vi "Subvi_Online_For_Offline_FBLDA_통합버전.vi"(0 "rate":dbl=500.0 caption="Rate" format="%0.2f", 1 "samples per channel":i32=25, 5 "Brain_data_source":dbl[][](array[numeric]) caption="EEG_Raw_Data" format="%0.3f", 7 "Target_Flash_Order":i64[][](array[numeric]), 8 "Value":T1, 9 "사용할 Parameter 갯수":i32=2, 10 "Weight":dbl[](array[numeric]), 11 "Path":path, 14 "Number":string, 16 "Matrix":T1, 17 "Channel selection":bool[](array[boolean])) -> (13 "LDA_Parameter":dbl[][](array[numeric]), 15 "EPR_발생_total":i16[](array[numeric]), 20 "output-0~8":i32, 22 "ERP_Parameters":dbl[][](array[numeric]))   [LabVIEW 2014]
uses:
  <vilib>/Analysis/Matrix/Datatypes/RealMatrix.ctl
  <vilib>/Analysis/3filter.llb/Filter Passband Type.ctl
  <vilib>/Analysis/baseanly.llb/Real A x B.vi
  <vilib>/Analysis/baseanly.llb/Mean (DBL).vi
  <vilib>/Analysis/3filter.llb/Butterworth Filter (DBL).vi
  <vilib>/Analysis/Matrix/Numeric/Conversions/Array To Matrix - RA.vi
  <vilib>/Analysis/Matrix/Numeric/Conversions/Array To Matrix - RA2.vi
  <vilib>/Analysis/Matrix/Numeric/Conversions/Matrix To Array - RM.vi
  <vilib>/Analysis/Matrix/Numeric/Multiply/Multiply - RM,RM.vi
  <vilib>/Analysis/Matrix/Numeric/Subtract/Subtract - RM,RM.vi
  <vilib>/Analysis/NI_AALBase.lvlib
  <vilib>/Analysis/Matrix/NI_Matrix.lvlib
  <vilib>/Utility/file.llb/Read From Spreadsheet File (DBL).vi
panel:
  out "최대값":dbl
  out "size(s)":i32[](array[numeric])
  out "A - B":T1
  out "Array 2":dbl[][](array[numeric])
  out "subarray":dbl[](array[numeric])
  out "Array":dbl[][](array[numeric])
  out "deleted portion":dbl[][](array[numeric])
  in  "LDA":path=path "C:/Users/Administrator/Desktop/공공복지안전사업연구-노수진/파일럿20130902/LDA_Matrix_Value.xls"
  out "#channel":i32
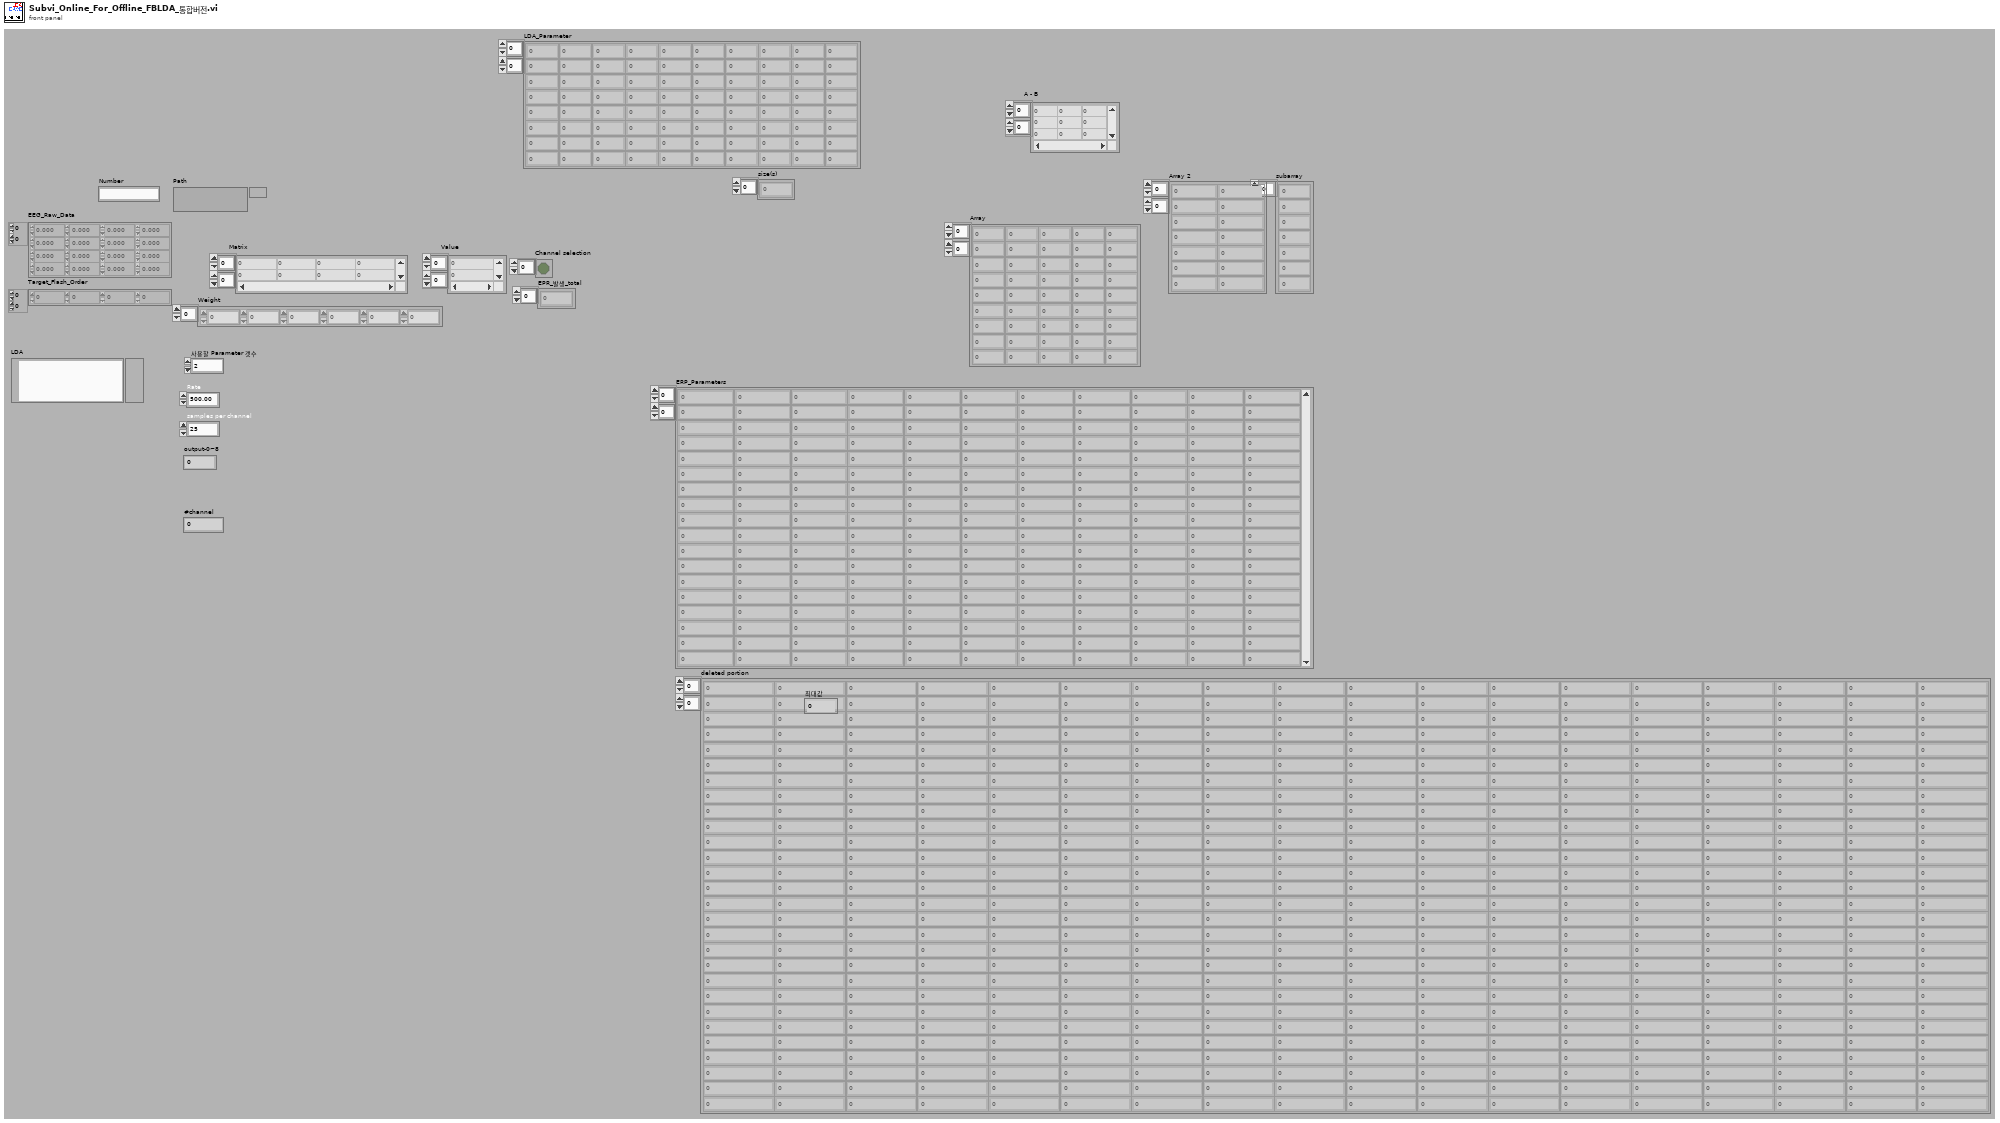
[diagram p1: front panel]
types:
  T1 = typedef "NI_Matrix.lvlib/RealMatrix.ctl" = dbl[][]
  T2 = typedef "NI_AALBase.lvlib/Filter Passband Type.ctl" = enum32{"Lowpass", "Highpass", "Bandpass", "Bandstop"}
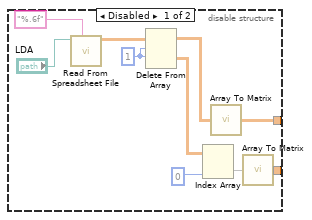
[diagram p3: hidden frame]
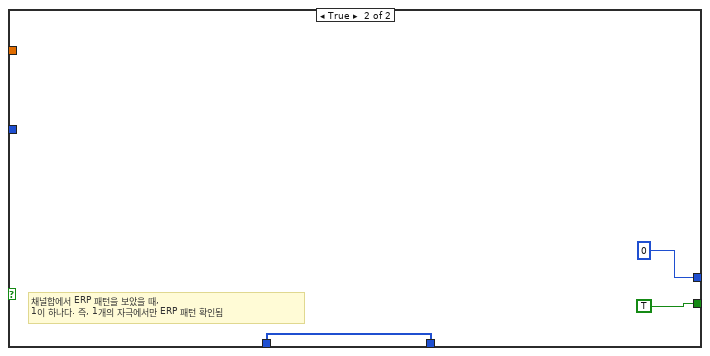
[diagram p4: hidden frame]
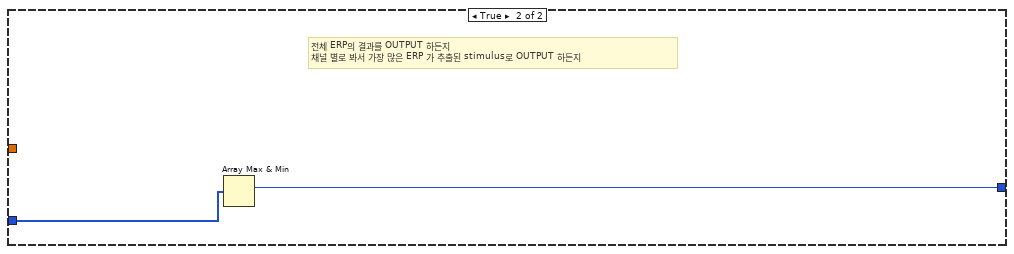
[diagram p5: hidden frame]
diagram:
  n1 = flat-sequence {
    tunnel: [w28] -> w23
    tunnel: [w52] -> w22
    tunnel: ["Target_Flash_Order"] -> w21
    tunnel: w23 -> [w52]
    tunnel: [w49] -> w20
    tunnel: w22 -> [w60]
    tunnel: w21 -> [w59]
    tunnel: w20 -> [w58]
    tunnel: [w53] -> w19
    tunnel: ["Weight"] -> w12
    tunnel: [w53] -> w1
    tunnel: w19 -> [w189]
    tunnel: [w191] -> w18
    tunnel: [w191] -> w17
    tunnel: [w191] -> w16
    tunnel: w12 -> [w186]
    tunnel: [w186] -> w11
    tunnel: [w180] -> w2
    tunnel: w1 -> [w180]
    tunnel: w18 -> [w228]
    tunnel: w17 -> [w234]
    tunnel: w16 -> [w221]
    tunnel: [w236] -> w15
    tunnel: w11 -> [w235]
    tunnel: [w235] -> w10
    tunnel: [w229] -> w9
    tunnel: [w219] -> w7
    tunnel: [w228] -> w5
    tunnel: [w227] -> w4
    tunnel: w2 -> [w220]
    tunnel: w15 -> [w257]
    tunnel: [w257] -> w14
    tunnel: w10 -> [_]
    tunnel: w9 -> [w260]
    tunnel: [w259] -> w8
    tunnel: w7 -> [w262]
    tunnel: [w262] -> w6
    tunnel: w5 -> [w261]
    tunnel: w4 -> [w258]
    tunnel: [w258] -> w3
    tunnel: [w285] -> w13
    tunnel: w14 -> [w286]
    tunnel: w8 -> [w284]
    tunnel: w6 -> [w283]
    tunnel: w3 -> [w282]
    tunnel: w13 -> [w307]
    frame #0 {
      n2 = Array Size(array="Brain_data_source") -> (size(s)=w29:i32[])
      n3 = Index Array(array=w29, index=1) -> (element=w31:i32)
      "#channel" <- w31
      n4 = for {
        N: w31 -> [_]
        tunnel: "Brain_data_source" -> [w36]
        shift-right: [w33] -> w25
        shift-left: dbl[][] [] ("Filtered X") -> [w34]
        tunnel: "Channel selection" -> [w32] mode=indexing
        i -> [w35]
        n5 = case shown="True" w32 {
          tunnel: w36 -> [_ w47]
          tunnel: w35 -> [_ w46]
          tunnel: w34 -> [w37 w40]
          tunnel: [w37 w39] -> w33
          frame False {
          }
          frame True {
            n6 = local read "rate"() -> (w41:dbl)
            n7 = Index Array(array=w47, index (col)=w46) -> (element=w45:dbl[])  [unwired: 1 in]
            n8 = call-poly <vilib>:"Butterworth Filter.vi"("filter type"=Filter_Passband_Type."Bandpass", "low cutoff freq: fl"=0.5, "high cutoff freq: fh"=30.0, "sampling freq: fs"=w41, "X"=w45) -> ("Filtered X"=w38:dbl[])  [unwired: 3 in, 1 out]
            n9 = Build Array (concatenate)(w40, w38) -> (w39:dbl[][])
          }
        }
      }
      n10 = Transpose 2D Array(2D array=w25) -> (transposed array=w28:dbl[][])
    }
    frame #1 {
      # "Bandpass per channel"
      # "20*9"
      n11 = Array Size(array="Target_Flash_Order") -> (size(s)=w51:i32[])
      n12 = Index Array(array=w51, index=1 ("인덱스")) -> (element=w49:i32)
    }
    frame #2 {
      (unwired) dbl[][] []
      (unwired) dbl[][] []
      n13 = for {
        N: w58 -> [_]
        tunnel: w60 -> [w74]
        tunnel: w59 -> [w73]
        shift-right: [w71] -> w53
        shift-left: dbl[][] [] -> [w70]
        shift-right: [w65] -> w55
        shift-left: dbl[][] [] -> [w64]
        tunnel: "Weight" -> [w63]
        i -> [w69]
        n14 = Index Array(array=w73, index (col)=w69) -> (element=w72:i64[])  [unwired: 1 in]
        n15 = flat-sequence {
          tunnel: w74 -> [w80]
          tunnel: w72 -> [w79]
          tunnel: [w78] -> w75
          tunnel: ["Path"] -> w68
          tunnel: ["Number"] -> w67
          tunnel: w75 -> [w141]
          tunnel: [w128] -> w62
          tunnel: w68 -> [_]
          tunnel: w67 -> [_]
          tunnel: [w120] -> w66
          tunnel: w63 -> [w131]
          frame #0 {
            # "10*600"
            # "Channel number"
            n16 = local read "samples per channel"() -> (w87:i32)
            n17 = local read "samples per channel"() -> (w86:i32)
            n18 = local read "rate"() -> (w89:dbl)
            n19 = Array Size(array=w80) -> (size(s)=w83:i32[])
            n20 = local read "rate"() -> (w91:dbl)
            n21 = Multiply(x=w89, y=0.2) -> (x*y=w93:dbl)
            n22 = Index Array(array=w83, index=1) -> (element=w85:i32)
            n23 = Add(x=w91, y=w93) -> (x+y=w92:dbl)
            n24 = Divide(x=w93, y=w87) -> (x/y=w90:dbl)
            n25 = Array Size(array=w79) -> (size(s)=w82:i32)
            n26 = for {
              N: w85 -> [_]
              tunnel: w86 -> [w94]
              tunnel: w92 -> [w105]
              shift-right: [w98] -> w78
              shift-left: dbl[][] [] -> [w100]
              tunnel: w82 -> [w99]
              tunnel: w80 -> [w97]
              tunnel: w79 -> [w96]
              tunnel: w90 -> [w95]
              i -> [w107]
              # "-20% ~ 100%: 1.2s epoch => 600 sample\ndim = 10*600 (ch# x 600 samp)"
              n27 = Initialize Array(0.0 ("element"), w105) -> (w104:dbl[])
              n28 = Index Array(array=w97, index (col)=w107) -> (element=w106:dbl[])  [unwired: 1 in]
              n29 = for {
                N: w99 -> [_]
                tunnel: w106 -> [w119]
                shift-right: [w116] -> w102
                shift-left: w104 -> [w117]
                tunnel: w105 -> [w115]
                tunnel: w96 -> [w113]
                tunnel: w95 -> [w111]
                tunnel: w94 -> [w109]
                i -> [w114]
                # "Average over each\nstimulus"
                # "20"
                n30 = Index Array(array=w113, index=w114) -> (element=w112:i64)
                n31 = Subtract(x=w112, y=w111) -> (x-y=w110:dbl)
                n32 = Multiply(x=w110, y=w109) -> (x*y=w108:dbl)
                n33 = Array Subset(array=w119, index=w108, length=w115) -> (w118:dbl[])
                n34 = Add(x=w118, y=w117) -> (x+y=w116:dbl[])
              }
              n35 = Divide(x=w102, y=w99) -> (x/y=w101:dbl[])
              n36 = Build Array (concatenate)(w100, w101) -> (w98:dbl[][])
            }
          }
          frame #1 {
            # "Weighted_Sum"
            # "epoch_size=600"
            # "250~450ms : P3 발생\n0~200 : N1 발생"
            # "10 + 1"
            n37 = Transpose 2D Array(2D array=w141) -> (transposed array=w129:dbl[][])
            n38 = Array Size(array=w129) -> (size(s)=w142:i32[])
            n39 = call-poly <vilib>:"Array To Matrix.vi"("Real 1D Array"=w131) -> ("Real Matrix (Column Vector)"=w137:T1)
            n40 = call-poly <vilib>:"Array To Matrix.vi"("Real 2D Array"=w129) -> ("Real Matrix"=w138:T1)
            n41 = Array Size(array=w129) -> (size(s)=w133:i32[])
            n42 = Index Array(array=w142, index #1=1 ("index"), index #2=0 ("인덱스")) -> (element #1=w139:i32)  [unwired: 1 out]
            n43 = Index Array(array=w133, index=0) -> (element=w132:i32)
            n44 = call-poly <vilib>:"A x B.vi"("B"=w137, "A"=w138) -> ("A x B"=w136:T1)  [unwired: 1 out]
            n45 = call-poly <vilib>:"Matrix To Array.vi"("Real Matrix"=w136) -> ("Real 2D Array"=w134:dbl[][])
            n46 = Increment(x=w139) -> (x+1=w127:i32)
            n47 = Reshape Array(w134, w132) -> (w130:dbl[])
            n48 = Insert Into Array(array=w129, index (col)=w139, new element=w130) -> (w122:dbl[][])  [unwired: 1 in]
            n49 = for {
              N: w127 -> [_]
              tunnel: w122 -> [w173]
              tunnel: [w151] -> w126 mode=indexing
              tunnel: [w150] -> w125 mode=indexing
              tunnel: [w149] -> w123 mode=indexing
              tunnel: [w148] -> w124 mode=indexing
              tunnel: [w147] -> _ mode=indexing
              shift-right: [w144] -> w120
              shift-left: dbl[][] [] -> [w146]
              i -> [w158]
              n50 = local read "rate"() -> (w172:dbl)
              n51 = Index Array(array=w173, index (col)=w158) -> (element=w163:dbl[])  [unwired: 1 in]
              n52 = Multiply(x=w172, y=0.2) -> (x*y=w170:dbl)
              n53 = Split 1D Array(array=w163, index=w170) -> (first subarray=w169:dbl[], second subarray=w154:dbl[])
              n54 = local read "rate"() -> (w166:dbl)
              n55 = call-poly <vilib>:"Mean.vi"("X"=w169) -> ("mean"=w168:dbl)  [unwired: 1 out]
              n56 = Multiply(x=w166, y=0.1) -> (x*y=w152:dbl)
              n57 = Subtract(x=w154, y=w168) -> (x-y=w145:dbl[])
              n58 = Divide(x=w166, y=w152) -> (x/y=w165:dbl)
              n59 = for {
                N: w165 -> [_]
                tunnel: w145 -> [w178]
                tunnel: [w179] -> w162 mode=indexing
                tunnel: w152 -> [w176]
                i -> [w175]
                n60 = Multiply(x=w175, y=w176) -> (x*y=w177:dbl)
                n61 = Array Subset(array=w178, index=w177, length=w176) -> (w174:dbl[])
                n62 = call-poly <vilib>:"Mean.vi"("X"=w174) -> ("mean"=w179:dbl)  [unwired: 1 out]
              }
              n63 = Build Array (concatenate)(w146, w145) -> (w144:dbl[][])
              n64 = Array Max & Min(array=w162) -> (max index (indices)=w157:i32)  [unwired: 3 out]
              n65 = Array Max & Min(array=w162) -> (min index (indices)=w156:i32)  [unwired: 3 out]
              n66 = Multiply(x=w157, y=w152) -> (x*y=w153:dbl)
              n67 = Multiply(x=w156, y=w152) -> (x*y=w160:dbl)
              n68 = Array Subset(array=w145, index=w153, length=w152) -> (w155:dbl[])
              n69 = Array Subset(array=w145, index=w160, length=w152) -> (w161:dbl[])
              n70 = Array Max & Min(array=w161) -> (min value=w149:dbl, min index (indices)=w159:i32)  [unwired: 2 out]
              n71 = Array Max & Min(array=w155) -> (max value=w151:dbl, max index (indices)=w164:i32)  [unwired: 2 out]
              n72 = Add(x=w164, y=w153) -> (x+y=w150:dbl)
              n73 = Add(x=w160, y=w159) -> (x+y=w148:dbl)
              n74 = Build Array(w151, w150, w149, w148) -> (w147:dbl[])
            }
            n75 = Build Array(w126, w125, w123, w124) -> (w128:dbl[][])
          }
        }
        n76 = Transpose 2D Array(2D array=w62) -> (transposed array=w61:dbl[][])
        n77 = Build Array (concatenate)(w64, w66) -> (w65:dbl[][])
        n78 = Build Array (concatenate)(w70, w61) -> (w71:dbl[][])
        "Array" <- w62
      }
      "ERP_Parameters" <- w53
      "LDA_Parameter" <- w55
    }
    frame #3 {
      # "여기 틀림"
      # "ERP_Parameter\n\n1. P3_Amp\n2. P3_Latency\n3. N1_Amp\n4. N1_Latency"
      n79 = disable-structure shown="Enabled" {
        disable-tunnel: [w198 "Matrix"] -> w183
        disable-tunnel: [w197 "Value"] -> w190
        frame Disabled {
          w200 = 1 ("인덱스 (행)")
          n80 = call-poly <vilib>:"Read From Spreadsheet File.vi"("format (%.3f)"="%.6f", "file path (dialog if empty)"="LDA") -> ("all rows"=w194:dbl[][])  [unwired: 5 in, 4 out]
          n81 = Delete From Array(array=w194, length=w200, index (row)=w200) -> (deleted portion=w203:dbl[][], array with subset deleted=w202:dbl[][])  [unwired: 1 in]
          n82 = Index Array(array=w203, index (col)=0 ("인덱스")) -> (element=w201:dbl[])  [unwired: 1 in]
          n83 = call-poly <vilib>:"Array To Matrix.vi"("Real 2D Array"=w202) -> ("Real Matrix"=w198:T1)
          n84 = call-poly <vilib>:"Array To Matrix.vi"("Real 1D Array"=w201) -> ("Real Matrix (Column Vector)"=w197:T1)
        }
        frame Enabled {
        }
      }
      n85 = Delete From Array(array=w189, length="사용할 Parameter 갯수", index (col)=0 ("비활성화된 인덱스 (열)")) -> (deleted portion=w188:dbl[][])  [unwired: 1 in, 1 out]
      "deleted portion" <- w188
      n86 = for {
        tunnel: w183 -> [w210]
        tunnel: w190 -> [w217]
        shift-right: [w215] -> w192
        shift-left: dbl[][] [] -> [w214]
        tunnel: w188 -> [w213] mode=indexing
        n87 = call-poly <vilib>:"Array To Matrix.vi"("Real 1D Array"=w213) -> ("Real Matrix (Column Vector)"=w211:T1)
        n88 = call-poly <vilib>:"Multiply.vi"("Real Matrix B"=w211, "Real Matrix A"=w210) -> ("A * B"=w212:T1)
        "A - B" <- w212
        n89 = call-poly <vilib>:"Subtract.vi"("Real Matrix B"=w217, "Real Matrix A"=w212) -> ("A - B"=w218:T1)
        n90 = call-poly <vilib>:"Matrix To Array.vi"("Real Matrix"=w218) -> ("Real 2D Array"=w216:dbl[][])
        n91 = Build Array (concatenate)(w214, w216) -> (w215:dbl[][])
      }
      "Array 2" <- w192
      n92 = Array Size(array=w183) -> (size(s)=→"size(s)":i32[])
      n93 = Index Array(array=w192, index (col)=0 ("비활성화된 인덱스 (열)")) -> (element=w184:dbl[])  [unwired: 1 in]
      "subarray" <- w184
      n94 = for {
        tunnel: w184 -> [w209] mode=indexing
        tunnel: [w208] -> w191 mode=indexing
        n95 = Greater?(x=w209, y=0.0) -> (0:w206:bool)
        n96 = Boolean To (0,1)(Boolean=w206) -> (0, 1=w208:i16)
      }
    }
    frame #4 {
      n97 = local read "#channel"() -> (w231:i32)
      n98 = Array Size(array=w234) -> (size(s)=w233:i32)
      n99 = Increment(x=w231) -> (x+1=w232:i32)
      n100 = Divide(x=w233, y=w232) -> (x/y=w227:dbl)
      n101 = Index Array(array=w220, index (col) #1=0 ("비활성화된 인덱스 (열)"), index (col) #2=2 ("인덱스 (열)")) -> (element #1=w223:dbl[], element #2=w226:dbl[])  [unwired: 2 in]
      n102 = for {
        N: w227 -> [_]
        tunnel: w232 -> [w255]
        tunnel: w231 -> [w253]
        tunnel: w221 -> [w252]
        shift-right: [w249] -> w229
        shift-left: i16[] [] -> [w250]
        i -> [w256]
        n103 = Multiply(x=w255, y=w256) -> (x*y=w254:i32)
        n104 = Add(x=w253, y=w254) -> (x+y=w248:i32)
        n105 = Index Array(array=w252, index=w248) -> (element=w251:i16)
        n106 = Build Array (concatenate)(w250, w251) -> (w249:i16[])
      }
      n107 = for {
        tunnel: w221 -> [w244] mode=indexing
        tunnel: w223 -> [w247] mode=indexing
        shift-right: [w245] -> w219
        shift-left: dbl[] [] -> [w246]
        tunnel: w226 -> [w243] mode=indexing
        n108 = Multiply(x=w244, y=w247) -> (x*y=w241:dbl)
        n109 = Multiply(x=w244, y=w243) -> (x*y=w239:dbl)
        n110 = Absolute Value(x=w239) -> (abs(x)=w242:dbl)
        n111 = Add(x=w241, y=w242) -> (x+y=w240:dbl)
        n112 = Build Array (concatenate)(w246, w240) -> (w245:dbl[])
      }
      n113 = Add Array Elements(numeric array=w229) -> (sum=w238:i16)
      n114 = Equal?(x=w238, y=i16 1) -> (x = y?=w236:bool)
      "EPR_발생_total" <- w221
    }
    frame #5 {
      # "#1> #2\n참에서는 참으로만\n참에서 거짓: 불가능\n거짓에서 참: 가능 (전체에선 단독 ERP가 안나왔지만 채널 별로 보니까 나옴)"
      # "#1"
      n115 = case shown="False" w257 {
        tunnel: [FALSE TRUE] -> _
        tunnel: [w267 0] -> _
        tunnel: [w266 w279] -> w259
        tunnel: w261 -> [w264 _]
        tunnel: w258 -> [w263 _]
        tunnel: w260 -> [_ w279]
        frame False {
          n116 = for {
            N: w263 -> [_]
            shift-right: [w272] -> w266
            shift-left: i16[] [] -> [w273]
            tunnel: w264 -> [w269]
            i -> [w278]
            # "9번 돌음\n채널의 1, 0 을 모두 더함"
            n117 = local read "#channel"() -> (w271:i32)
            n118 = Add(x=1, y=w271) -> (x+y=w276:i32)
            n119 = Multiply(x=w278, y=w276) -> (x*y=w275:i32)
            n120 = Array Subset(array=w269, index=w275, length=w271) -> (w270:i16[])
            n121 = Add Array Elements(numeric array=w270) -> (sum=w274:i16)
            n122 = Build Array (concatenate)(w273, w274) -> (w272:i16[])
          }
          n123 = Array Max & Min(array=w266) -> (max value=w267:i16)  [unwired: 3 out]
          "최대값" <- w267
        }
        frame True {
          # "채널합에서 ERP 패턴을 보았을 때,\n1이 하나다. 즉, 1개의 자극에서만 ERP 패턴 확인됨"
        }
      }
    }
    frame #6 {
      # "#2"
      n124 = case shown="False" w286 {
        tunnel: [w292 w306] -> w285
        tunnel: w284 -> [w290 w305]
        tunnel: w283 -> [w289 _]
        tunnel: w282 -> [w291 _]
        frame False {
          n125 = for {
            N: w291 -> [_]
            tunnel: w290 -> [w299] mode=indexing
            tunnel: w289 -> [w298]
            shift-right: [w294] -> w287
            shift-left: dbl[] [] -> [w293]
            i -> [w297]
            n126 = local read "#channel"() -> (w296:i32)
            n127 = Add(x=1, y=w296) -> (x+y=w301:i32)
            n128 = Multiply(x=w297, y=w301) -> (x*y=w302:i32)
            n129 = Array Subset(array=w298, index=w302, length=w296) -> (w303:dbl[])
            n130 = Add Array Elements(numeric array=w303) -> (sum=w304:dbl)
            n131 = Divide(x=w304, y=w299) -> (x/y=w295:dbl)
            n132 = Build Array (concatenate)(w293, w295) -> (w294:dbl[])
          }
          n133 = Array Max & Min(array=w287) -> (max index (indices)=w292:i32)  [unwired: 3 out]
        }
        frame True {
          # "전체 ERP의 결과를 OUTPUT 하든지\n채널 별로 봐서 가장 많은 ERP 가 추출된 stimulus로 OUTPUT 하든지"
          n134 = Array Max & Min(array=w305) -> (max index (indices)=w306:i32)  [unwired: 3 out]
        }
      }
    }
    frame #7 {
      "output-0~8" <- w307
    }
  }
